vi "FTW-Time-Display-Elapsed.vi"(1 "Format":T1=enum."Human Estimate", 3 "Elapsed Time (msec)":u32 format="%06dmsec") -> (0 "Elapsed Time":string)   [LabVIEW 2015]
uses:
  FTW-Time-DisplayFormat-Elapsed.ctl
panel:
  # "Inputs"
  # "Outputs"
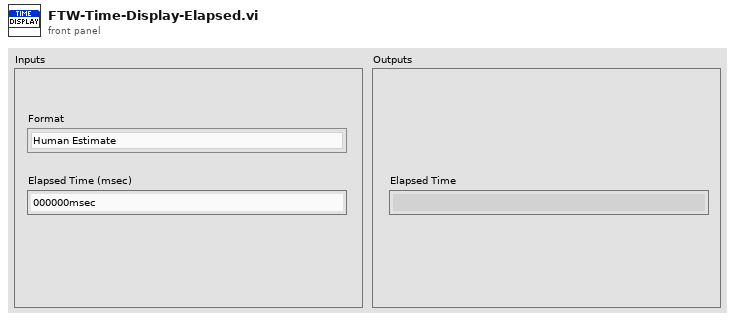
[diagram p1: front panel]
types:
  T1 = typedef "FTW-Time-DisplayFormat-Elapsed.ctl" = enum16{"HH:MM:SS.sss", "HH:MM:SS", "000000msec", "0msec", "0000.00sec", "0.000sec", "0sec", "0.00min", "Human Estimate"}
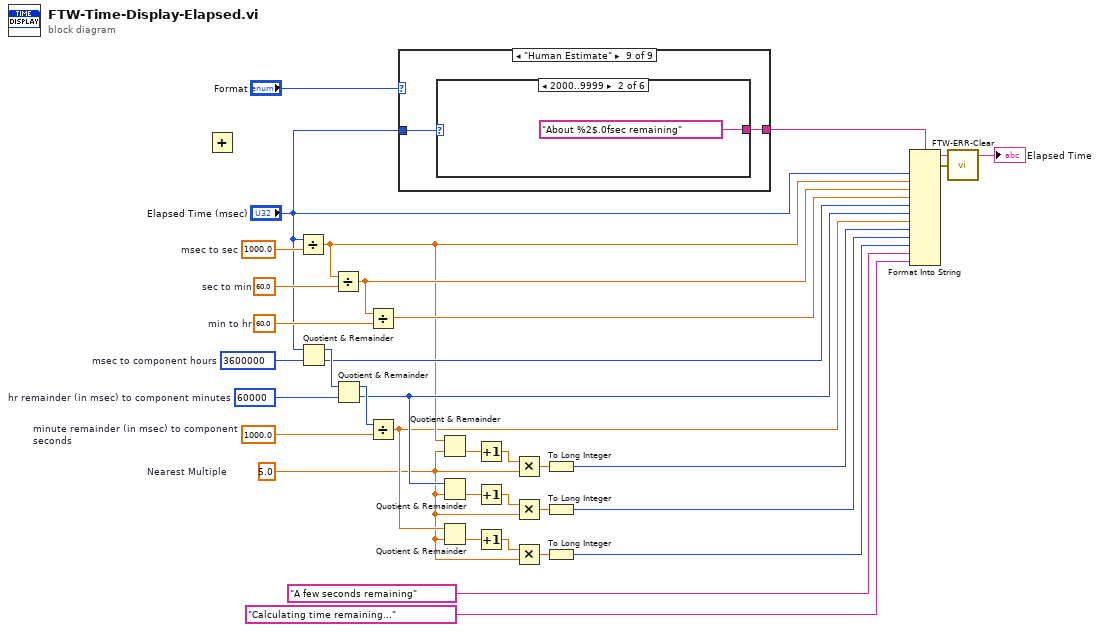
[diagram p0: block diagram]
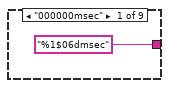
[diagram p2: hidden frame]
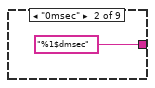
[diagram p3: hidden frame]
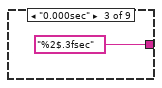
[diagram p4: hidden frame]
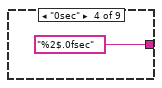
[diagram p5: hidden frame]
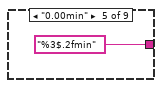
[diagram p6: hidden frame]
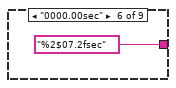
[diagram p7: hidden frame]
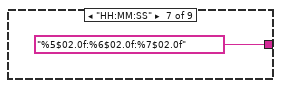
[diagram p8: hidden frame]
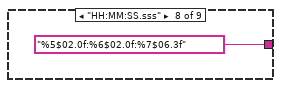
[diagram p9: hidden frame]
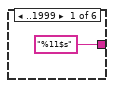
[diagram p10: hidden frame]
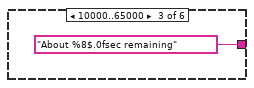
[diagram p11: hidden frame]
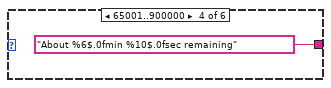
[diagram p12: hidden frame]
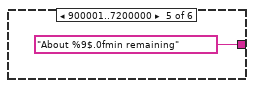
[diagram p13: hidden frame]
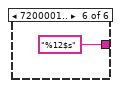
[diagram p14: hidden frame]
diagram:
  w4 = 5.0  # Nearest Multiple
  w22 = 1000.0  # minute remainder (in msec) to component seconds
  w25 = u32 3600000  # msec to component hours
  w26 = u32 60000  # hr remainder (in msec) to component minutes
  w30 = 60.0  # min to hr
  w31 = 60.0  # sec to min
  w32 = 1000.0  # msec to sec
  n1 = Add() -> ()  [unwired: 2 in, 1 out]
  n2 = Divide(x="Elapsed Time (msec)", y=w32) -> (x/y=w6:dbl)
  n3 = Quotient & Remainder(x="Elapsed Time (msec)", y=w25) -> (x-y*floor(x/y)=w24:u32, floor(x/y)=w21:u32)
  n4 = Divide(x=w6, y=w31) -> (x/y=w29:dbl)
  n5 = Quotient & Remainder(x=w24, y=w26) -> (x-y*floor(x/y)=w23:u32, floor(x/y)=w11:u32)
  n6 = Divide(x=w29, y=w30) -> (x/y=w28:dbl)
  n7 = Divide(x=w23, y=w22) -> (x/y=w5:dbl)
  n8 = case shown="\"Human Estimate\"" "Format" {
    tunnel: ["%1$06dmsec" ("format string") "%1$dmsec" ("format string") "%2$.3fsec" ("format string") "%2$.0fsec" ("format string") "%3$.2fmin" ("format string") "%2$07.2fsec" ("format string") "%5$02.0f:%6$02.0f:%7$02.0f" ("format string") "%5$02.0f:%6$02.0f:%7$06.3f" ("format string") w44] -> w27
    tunnel: "Elapsed Time (msec)" -> [_ _ _ _ _ _ _ _ w43]
    frame "000000msec" {
    }
    frame "0msec" {
    }
    frame "0.000sec" {
    }
    frame "0sec" {
    }
    frame "0.00min" {
    }
    frame "0000.00sec" {
    }
    frame "HH:MM:SS" {
    }
    frame "HH:MM:SS.sss" {
    }
    frame "Human Estimate" {
      n9 = case shown="2000..9999" w43 {
        tunnel: ["%11$s" ("format string") "About %2$.0fsec remaining" ("format string") "About %8$.0fsec remaining" ("format string") "About %6$.0fmin %10$.0fsec remaining" ("format string") "About %9$.0fmin remaining" ("format string") "%12$s" ("format string")] -> w44
        frame ..1999 {
        }
        frame 2000..9999 {
        }
        frame 10000..65000 {
        }
        frame 65001..900000 {
        }
        frame 900001..7200000 {
        }
        frame 7200001.. {
        }
      }
    }
  }
  n10 = Quotient & Remainder(x=w6, y=w4) -> (floor(x/y)=w19:dbl)  [unwired: 1 out]
  n11 = Quotient & Remainder(x=w11, y=w4) -> (floor(x/y)=w13:dbl)  [unwired: 1 out]
  n12 = Quotient & Remainder(x=w5, y=w4) -> (floor(x/y)=w10:dbl)  [unwired: 1 out]
  n13 = Increment(x=w19) -> (x+1=w17:dbl)
  n14 = Increment(x=w13) -> (x+1=w15:dbl)
  n15 = Increment(x=w10) -> (x+1=w8:dbl)
  n16 = Multiply(x=w17, y=w4) -> (x*y=w18:dbl)
  n17 = Multiply(x=w15, y=w4) -> (x*y=w14:dbl)
  n18 = Multiply(x=w8, y=w4) -> (x*y=w9:dbl)
  n19 = To Long Integer(number=w18) -> (32bit integer=w16:i32)
  n20 = To Long Integer(number=w14) -> (32bit integer=w12:i32)
  n21 = To Long Integer(number=w9) -> (32bit integer=w7:i32)
  n22 = Format Into String(format string=w27, "Elapsed Time (msec)", w6, w29, w28, w21, w11, w5, w16, w12, w7, "A few seconds remaining", "Calculating time remaining...") -> (resulting string=→"Elapsed Time":string, error out=w20:errorcluster)  [unwired: 2 in]
  n23 = call "FTW-ERR-Clear.vi"("error to snuff"=w20) -> ()  [unwired: 1 out]
